vi "WAIT_FOR_GUN.vi"(7 "arguments":string[](array[string]), 8 "dt":i32, 9 "Reinit":bool, 10 "bus_inputs":T1, 11 "bus_state":T2) -> (1 "Done":bool, 2 "bus_inputs out":T1, 3 "bus_state out":T2)   [LabVIEW 2013]
uses:
  structures/bus_state.ctl
  structures/bus_state_drivetrain.ctl
  structures/bus_state_collector.ctl
  collector/collector_shot_cal.ctl
  structures/bus_inputs.ctl
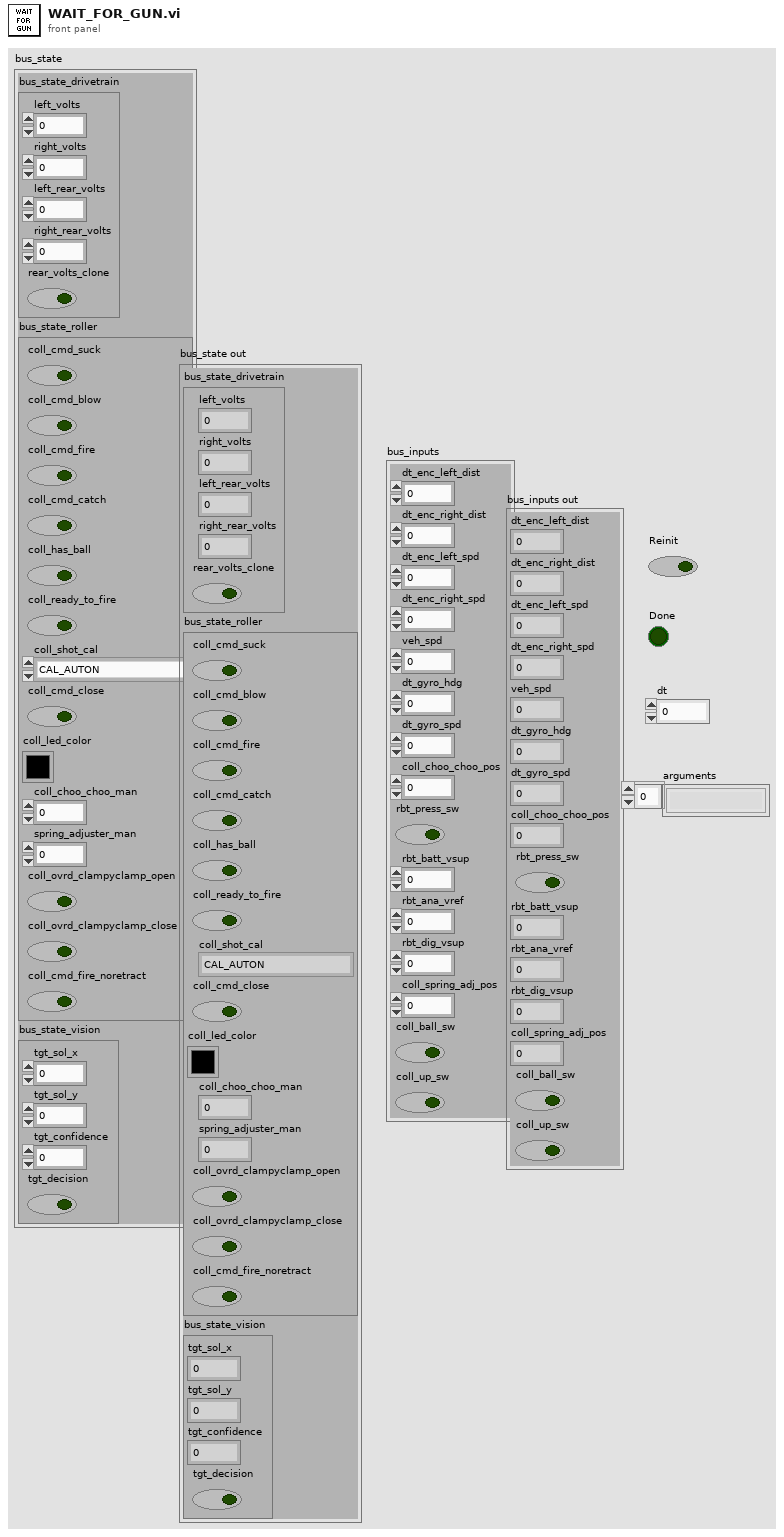
[diagram p1: front panel]
types:
  T1 = typedef "bus_inputs.ctl" = cluster{"dt_enc_left_dist":sgl, "dt_enc_right_dist":sgl, "dt_enc_left_spd":sgl, "dt_enc_right_spd":sgl, "veh_spd":sgl, "dt_gyro_hdg":sgl, "dt_gyro_spd":sgl, "coll_choo_choo_pos":sgl, "rbt_press_sw":bool, "rbt_batt_vsup":sgl, "rbt_ana_vref":dbl, "rbt_dig_vsup":dbl, "coll_spring_adj_pos":sgl, "coll_ball_sw":bool, "coll_up_sw":bool}
  T2 = typedef "bus_state.ctl" = cluster{"bus_state_drivetrain":T3, "bus_state_roller":T4, "bus_state_vision":cluster{"tgt_sol_x":dbl, "tgt_sol_y":dbl, "tgt_confidence":dbl, "tgt_decision":bool}}
  T3 = typedef "bus_state_drivetrain.ctl" = cluster{"left_volts":sgl, "right_volts":sgl, "left_rear_volts":sgl, "right_rear_volts":sgl, "rear_volts_clone":bool}
  T4 = typedef "bus_state_collector.ctl" = cluster{"coll_cmd_suck":bool, "coll_cmd_blow":bool, "coll_cmd_fire":bool, "coll_cmd_catch":bool, "coll_has_ball":bool, "coll_ready_to_fire":bool, "coll_shot_cal":T5, "coll_cmd_close":bool, "coll_led_color":u32, "coll_choo_choo_man":sgl, "spring_adjuster_man":sgl, "coll_ovrd_clampyclamp_open":bool, "coll_ovrd_clampyclamp_close":bool, "coll_cmd_fire_noretract":bool}
  T5 = typedef "collector_shot_cal.ctl" = enum16{"CAL_AUTON", "CAL_CLOSE", "CAL_MID", "CAL_FAR", "NOT_SAFE_TO_ACTUATE"}
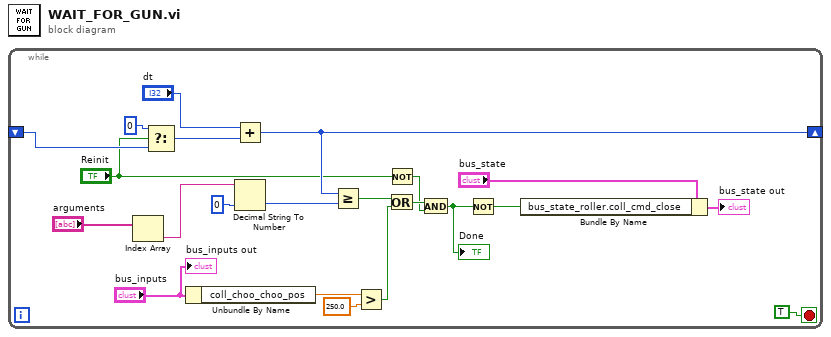
[diagram p0: block diagram]
diagram:
  n1 = while {
    shift-right: [w15] -> _
    shift-left: _ -> [w18]
    stop <- TRUE stop-if-true
    n2 = Index Array(array="arguments") -> (element=w21:string)  [unwired: 1 in]
    n3 = Select(t=0, s="Reinit", f=w18) -> (s? t:f=w16:i32)
    n4 = Unbundle By Name("bus_inputs") -> ("coll_choo_choo_pos"=w11:sgl)
    n5 = Add(x="dt", y=w16) -> (x+y=w15:i32)
    n6 = Decimal String To Number(string=w21, default (0L)=0 ("default (0 I32)")) -> (number=w13:i32)  [unwired: 1 in, 1 out]
    n7 = Greater Or Equal?(x=w15, y=w13) -> (x >= y?=w9:bool)
    n8 = Greater?(x=w11, y=250.0) -> (0:w8:bool)
    n9 = Not(x="Reinit") -> (.not. x?=w2:bool)
    n10 = Or(x=w9, y=w8) -> (x .or. y?=w4:bool)
    n11 = And(x=w4, y=w2) -> (x .and. y?=w3:bool)
    "Done" <- w3
    n12 = Not(x=w3) -> (.not. x?=w5:bool)
    n13 = Bundle By Name(cluster="bus_state", "bus_state_roller.coll_cmd_close"=w5) -> (→"bus_state out":T2)
    "bus_inputs out" <- "bus_inputs"
  }
